vi "clone.vi"(0 "reference":refnum<class "InterfaceNode.lvclass">, 5 "error in (no error)":errorcluster) -> (14 "reference out":refnum<class "InterfaceNode.lvclass">, 15 "clonedInterfaceNode":refnum<class "AbstractNode.lvclass">, 19 "error out":errorcluster)   [LabVIEW 2020, in "InterfaceNode.lvclass"]
doc: "public Object clone()"
uses:
  <resource>/Framework/Providers/Open_GDS/UML/InterfaceNode_class/InterfaceNode.lvclass
  C:/Program Files (x86)/National Instruments/LabVIEW 2020/resource/Framework/Providers/Open_GDS/UML/RectangularNode_class/RectangularNode.lvclass
  C:/Program Files (x86)/National Instruments/LabVIEW 2020/resource/Framework/Providers/Open_GDS/UML/ClassNode_class/ClassNode.lvclass
  C:/Program Files (x86)/National Instruments/LabVIEW 2020/resource/Framework/Providers/Open_GDS/UML/AbstractNode_class/AbstractNode.lvclass
  <resource>/Framework/Providers/Open_GDS/UML/AbstractNode_class/AbstractNode.lvclass
  <resource>/Framework/Providers/Open_GDS/UML/MultiLineString_class/MultiLineString.lvclass
  <resource>/Framework/Providers/Open_GDS/UML/ClassNode_class/ClassNode.lvclass
  <resource>/Framework/Providers/Open_GDS/UML/RectangularNode_class/RectangularNode.lvclass
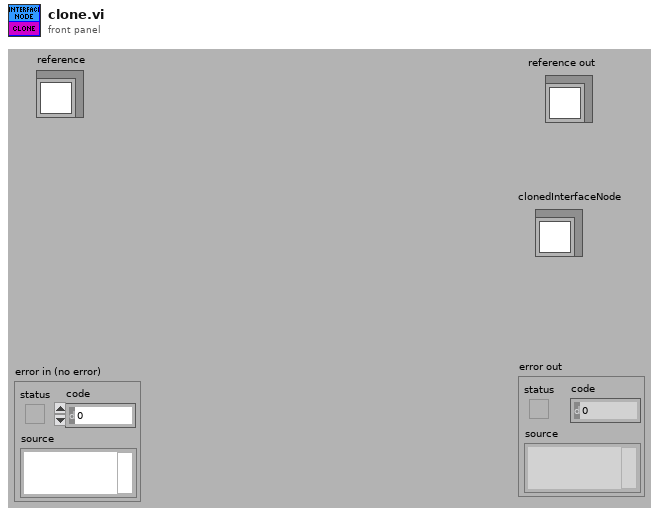
[diagram p1: front panel]
types:
  T1 = typedef "RectangularNode.lvclass/ObjectAttributes.ctl" = cluster{"bounds":T2}
  T2 = typedef "Rectangle Rectangle2D.ctl" = cluster{"x":dbl, "y":dbl, "width":dbl, "height":dbl}
  T3 = typedef "ClassNode.lvclass/ObjectAttributes.ctl" = cluster{"midHeight":dbl, "botHeight":dbl, "name":refnum<class "MultiLineString.lvclass">, "attributes":refnum<class "MultiLineString.lvclass">, "methods":refnum<class "MultiLineString.lvclass">, "DEFAULT_COMPARTMENT_HEIGHT":i32, "DEFAULT_WIDTH":i32, "DEFAULT_HEIGHT":i32, "showMethods":bool, "showAttributes":bool, "ClassPath":path}
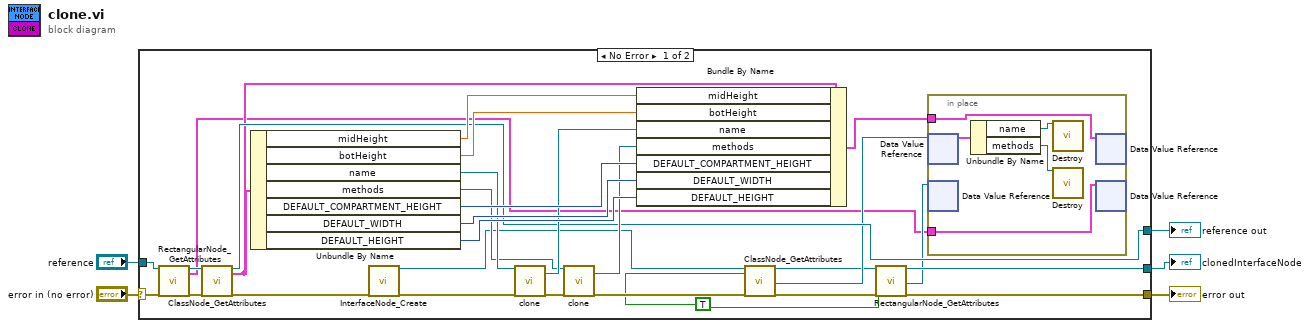
[diagram p0: block diagram]
diagram:
  n1 = case shown="No Error" "error in (no error)" {
    selector: "error in (no error)" -> [w34 w40]
    tunnel: "reference" -> [w13 w41]
    tunnel: [w11 w40] -> w4
    tunnel: [w21 w41] -> w3
    tunnel: [w9 _] -> w1
    frame No Error {
      w6 = TRUE ("OnlyGetDvrReference(False)")
      n2 = call <resource>:"RectangularNode_GetAttributes.vi"("reference in"=w13, "error in (no error)"=w34) -> ("reference out"=w12:refnum<class "InterfaceNode.lvclass">, "Data"=w7:T1, "error out"=w14:errorcluster)  [unwired: 14 in, 1 out]
      n3 = call <resource>:"ClassNode_GetAttributes.vi"("reference in"=w12, "error in (no error)"=w14) -> ("reference out"=w21:refnum<class "InterfaceNode.lvclass">, "Data"=w18:T3, "error out"=w20:errorcluster)  [unwired: 14 in, 1 out]
      n4 = Unbundle By Name(w18) -> ("midHeight"=w33:dbl, "botHeight"=w32:dbl, "name"=w27:refnum<class "MultiLineString.lvclass">, "methods"=w25:refnum<class "MultiLineString.lvclass">, "DEFAULT_COMPARTMENT_HEIGHT"=w31:i32, "DEFAULT_WIDTH"=w30:i32, "DEFAULT_HEIGHT"=w29:i32)
      n5 = call <resource>:"InterfaceNode_Create.vi"("error in (no error)"=w20) -> ("reference out"=w19:refnum<class "InterfaceNode.lvclass">, "error out"=w28:errorcluster)  [unwired: 17 in]
      n6 = call-dynamic "clone.vi"("reference"=w27, "error in (no error)"=w28) -> ("clonedMultiLineString"=w26:refnum<class "MultiLineString.lvclass">, "error out"=w22:errorcluster)  [unwired: 15 in, 1 out]
      n7 = call-dynamic "clone.vi"("reference"=w25, "error in (no error)"=w22) -> ("clonedMultiLineString"=w24:refnum<class "MultiLineString.lvclass">, "error out"=w23:errorcluster)  [unwired: 15 in, 1 out]
      n8 = Bundle By Name(cluster=w18, "midHeight"=w33, "botHeight"=w32, "name"=w26, "methods"=w24, "DEFAULT_COMPARTMENT_HEIGHT"=w31, "DEFAULT_WIDTH"=w30, "DEFAULT_HEIGHT"=w29) -> (w15:T3)
      n9 = call <resource>:"ClassNode_GetAttributes.vi"("reference in"=w19, "OnlyGetDvrReference(False)"=w6, "error in (no error)"=w23) -> ("reference out"=w10:refnum<class "InterfaceNode.lvclass">, "DataRef"=w16:refnum<data-value>, "error out"=w17:errorcluster)  [unwired: 13 in, 1 out]
      n10 = call <resource>:"RectangularNode_GetAttributes.vi"("reference in"=w10, "OnlyGetDvrReference(False)"=w6, "error in (no error)"=w17) -> ("reference out"=w9:refnum<class "InterfaceNode.lvclass">, "DataRef"=w8:refnum<data-value>, "error out"=w11:errorcluster)  [unwired: 13 in, 1 out]
      n11 = in-place {
        in-place-border: w15 -> [w39]
        in-place-border: w7 -> [w35]
        n12 = in-place-dvr #1(w16) -> (w37:T3)  [unwired: 1 out]
        n13 = in-place-dvr #2(w8) -> ()  [unwired: 2 out]
        n14 = Unbundle By Name(w37) -> ("name"=w38:refnum<class "MultiLineString.lvclass">, "methods"=w36:refnum<class "MultiLineString.lvclass">)
        n15 = call-dynamic "Destroy.vi"("reference"=w38) -> ()  [unwired: 17 in, 2 out]
        n16 = call-dynamic "Destroy.vi"("reference"=w36) -> ()  [unwired: 17 in, 2 out]
        n17 = in-place-dvr #1(w39) -> ()  [unwired: 2 out]
        n18 = in-place-dvr #2(w35) -> ()  [unwired: 2 out]
      }
    }
    frame Error {
    }
  }
  "reference out" <- w3
  "error out" <- w4
  "clonedInterfaceNode" <- w1
